vi "Update MSG.vi"(8 "error in (no error)":errorcluster, 10 "Update MSG":string, 11 "ENG Actor in":refnum<class "ENG Actor.lvclass">) -> (0 "error out":errorcluster, 3 "ENG Actor out":refnum<class "ENG Actor.lvclass">)   [LabVIEW 2020, in "ENG Actor.lvlib" / "ENG Actor.lvclass"]
uses:
  ENG Actor.lvclass
  ENG Actor.lvclass/ENG Actor.ctl
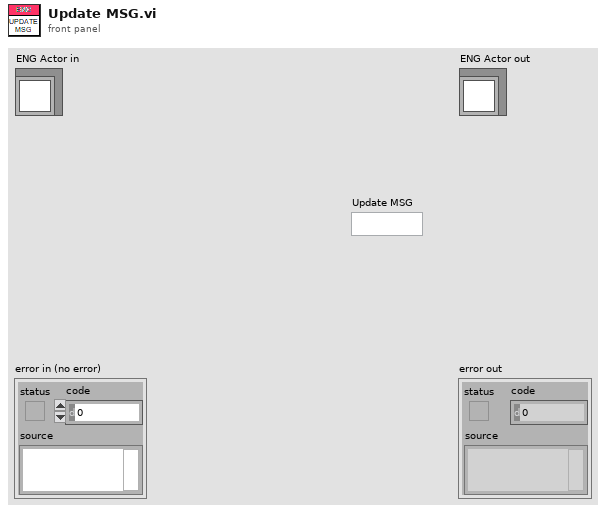
[diagram p1: front panel]
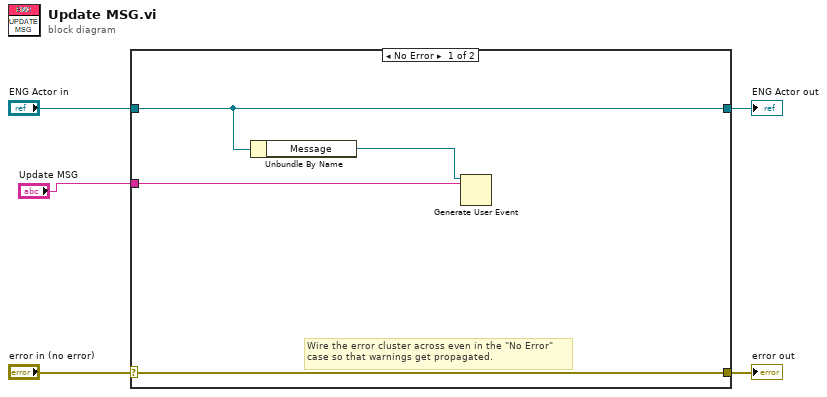
[diagram p0: block diagram]
diagram:
  n1 = case shown="No Error" "error in (no error)" {
    selector: "error in (no error)" -> [w9 w11]
    tunnel: [w9 w11] -> w4
    tunnel: [w6 w10] -> w2
    tunnel: "ENG Actor in" -> [w6 w10]
    tunnel: "Update MSG" -> [w7 _]
    frame No Error {
      # "Wire the error cluster across even in the \"No Error\"\ncase so that warnings get propagated."
      n2 = Unbundle By Name(w6) -> ("Message"=w8:refnum<user-event>)
      n3 = Generate User Event(user event=w8, event data cluster=w7) -> ()  [unwired: 2 in, 2 out]
    }
    frame Error {
    }
  }
  "error out" <- w4
  "ENG Actor out" <- w2
